vi "getStandardFolderName.vi"(4 "Name in":string) -> (1 "Folder name out":string)   [LabVIEW 2022 SP3, in "openDAQ.lvlib" / "daqUtils.lvlib" / "Tree.lvlib"]
uses:
  Tree.lvlib
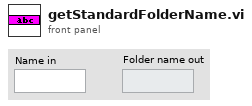
[diagram p1: front panel]
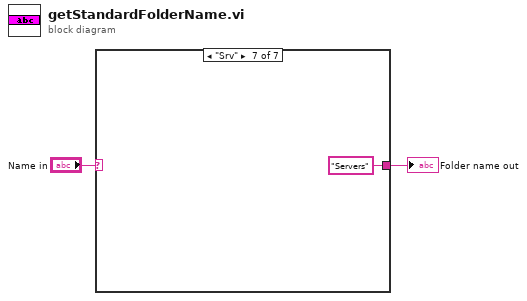
[diagram p0: block diagram]
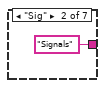
[diagram p3: hidden frame]
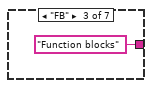
[diagram p4: hidden frame]
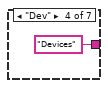
[diagram p5: hidden frame]
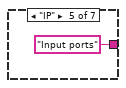
[diagram p6: hidden frame]
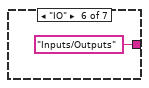
[diagram p7: hidden frame]
diagram:
  n1 = case shown="\"Srv\"" "Name in" {
    selector: "Name in" -> [w3 _ _ _ _ _ _]
    tunnel: [w3 "Signals" "Function blocks" "Devices" "Input ports" "Inputs/Outputs" "Servers"] -> w1
    frame Default {
    }
    frame "Sig" {
    }
    frame "FB" {
    }
    frame "Dev" {
    }
    frame "IP" {
    }
    frame "IO" {
    }
    frame "Srv" {
    }
  }
  "Folder name out" <- w1
